vi "BRig_RT_comm_tcp_write_RTwrite.vi"(8 "input_error":errorcluster, 10 "input_packet":string, 11 "input_hTCP":refnum<k5>) -> (0 "output_error":errorcluster, 1 "output_I_NotDisconnected":bool, 2 "output_I_write":bool, 3 "output_hTCP":refnum<k5>)   [LabVIEW 2014]
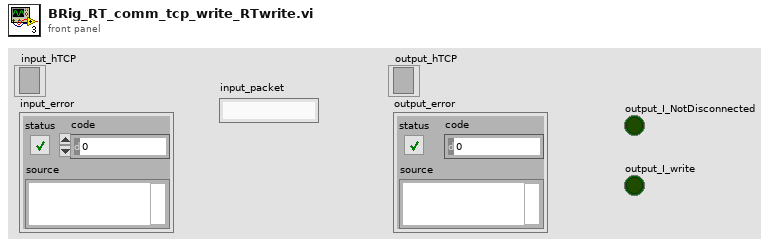
[diagram p1: front panel]
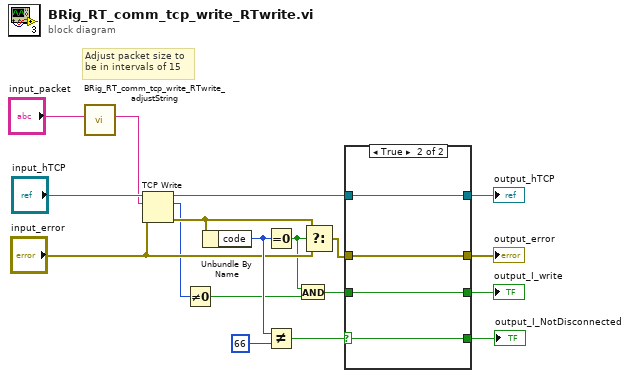
[diagram p0: block diagram]
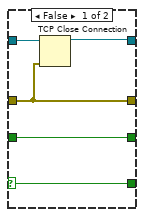
[diagram p2: hidden frame]
diagram:
  # "Adjust packet size to\nbe in intervals of 15"
  n1 = call "BRig_RT_comm_tcp_write_RTwrite_adjustString.vi"("input_packet"="input_packet") -> ("output_packet"=w1:string)  [unwired: 10 in]
  n2 = TCP Write(connection ID="input_hTCP", data in=w1, error in (no error)="input_error") -> (connection ID out=w10:refnum<k5>, bytes written=w14:i32, error out=w17:errorcluster)  [unwired: 1 out]
  n3 = Not Equal To 0?(x=w14) -> (x != 0?=w13:bool)
  n4 = Unbundle By Name(w17) -> ("code"=w16:i32)
  n5 = Equal To 0?(x=w16) -> (x = 0?=w12:bool)
  n6 = Not Equal?(x=w16, y=66) -> (x != y?=w6:bool)
  n7 = And(x=w12, y=w13) -> (x .and. y?=w4:bool)
  n8 = Select(t=w17, s=w12, f="input_error") -> (s? t:f=w7:errorcluster)
  n9 = case shown="True" w6 {
    selector: w6 -> [w20 w27]
    tunnel: w10 -> [w23 w24]
    tunnel: [w22 w24] -> w9
    tunnel: [w19 w25] -> w8
    tunnel: w7 -> [w19 w25]
    tunnel: [w20 w27] -> w5
    tunnel: w4 -> [w21 w26]
    tunnel: [w21 w26] -> w3
    frame False {
      n10 = TCP Close Connection(connection ID=w23, error in (no error)=w19) -> (connection ID out=w22:refnum<k5>)  [unwired: 1 in, 1 out]
    }
    frame True {
    }
  }
  "output_hTCP" <- w9
  "output_error" <- w8
  "output_I_write" <- w3
  "output_I_NotDisconnected" <- w5
